vi "Parse ERD Read Expected Data (Rev 2 API).vi"(0 "ERD Read Data In":T1 {"ERD Number" format="%.0x"}, 5 "Request ID":string, 11 "Error In":errorcluster) -> (8 "Expected Data":string, 15 "Error Out":errorcluster)   [LabVIEW 2023, in "GEA2_Toolkit.lvlib"]
uses:
  library/GEA2_Toolkit.lvlib
  type defs/ERD Read Data In.ctl
  type defs/Data Type.ctl
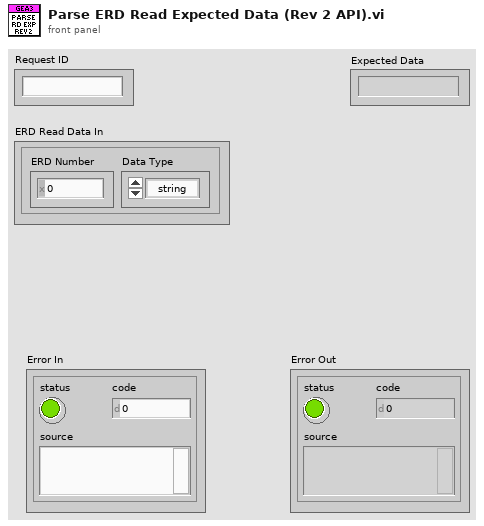
[diagram p1: front panel]
types:
  T1 = typedef "GEA2_Toolkit.lvlib/ERD Read Data In.ctl" = cluster{"ERD Number":u16, "Data Type":T2}
  T2 = typedef "GEA2_Toolkit.lvlib/Data Type.ctl" = enum16{"string", "boolean", "uint8_t", "uint16_t", "uint32_t", "uint64_t", "int8_t", "int16_t", "int32_t", "int64_t"}
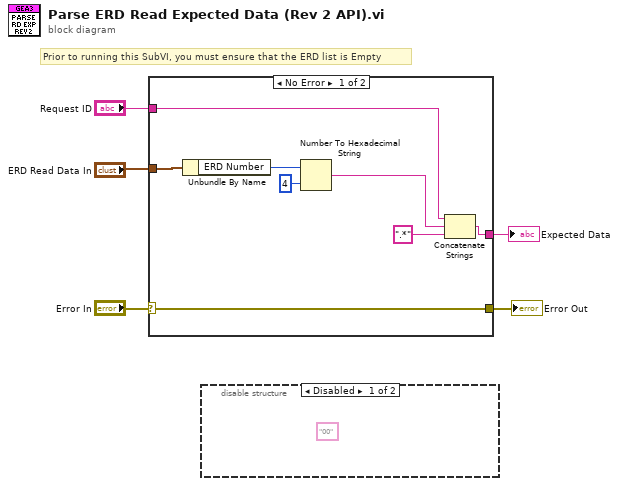
[diagram p0: block diagram]
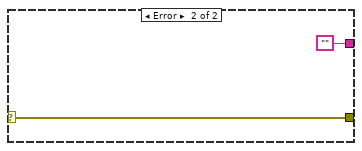
[diagram p3: hidden frame]
diagram:
  # "Prior to running this SubVI, you must ensure that the ERD list is Empty"
  n1 = case shown="No Error" "Error In" {
    selector: "Error In" -> [w12 w15]
    tunnel: [w13 ""] -> w5
    tunnel: "ERD Read Data In" -> [w7 _]
    tunnel: [w12 w15] -> w3
    tunnel: "Request ID" -> [w6 _]
    frame No Error {
      n2 = Unbundle By Name(w7) -> ("ERD Number"=w10:u16)
      n3 = Number To Hexadecimal String(1:i16 4 ("width (-)"), 2:w10) -> (0:w9:string)
      n4 = Concatenate Strings(w6, w9, ".*") -> (w13:string)
    }
    frame Error {
    }
  }
  "Expected Data" <- w5
  "Error Out" <- w3
  n5 = disable-structure shown="Disabled" {
    frame Disabled {
      (unwired) "00" ("string")
    }
    frame Enabled {
    }
  }
